vi "Write.Lookup.vi"(8 "error in":errorcluster, 10 "Name":string, 11 "Data Access API in":refnum<class "Plugin Data Access Engine.lvclass">) -> (0 "error out":errorcluster, 1 "Initial Values":dbl[](array[numeric]), 2 "Ref":T1, 3 "Data Access API out":refnum<class "Plugin Data Access Engine.lvclass">)   [LabVIEW 2023, in "Plugin Data Access Engine.lvlib" / "Plugin Data Access Engine.lvclass"]
uses:
  Plugin Data Access Engine.lvclass
  Types/Write.DVR.ctl
  Access Type Classes/Write/Write.lvclass
  Plugin Data Access Engine.lvclass/Plugin Data Access Engine.ctl
  Types/VS Channel Group Type.ctl
  Access Type Classes/Write/Write.lvclass/Write.ctl
  Access Type Classes/Write/Write.ReadValues.vi
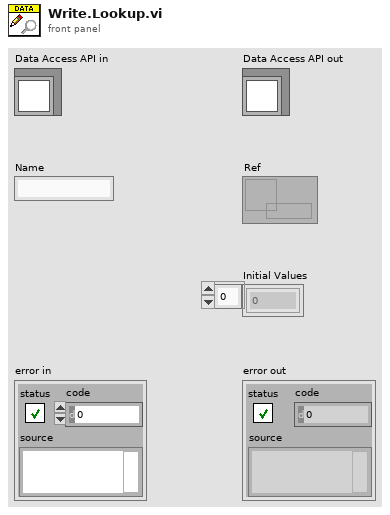
[diagram p1: front panel]
types:
  T1 = typedef "Plugin Data Access Engine.lvlib/Plugin Data Access Engine.lvclass/Write.DVR.ctl" = refnum<data-value>
  T2 = typedef "Plugin Data Access Engine.lvlib/Plugin Data Access Engine.lvclass/VS Channel Group Type.ctl" = enum16{"Output/Write", "Input/Read", "Input/ReadWrite"}
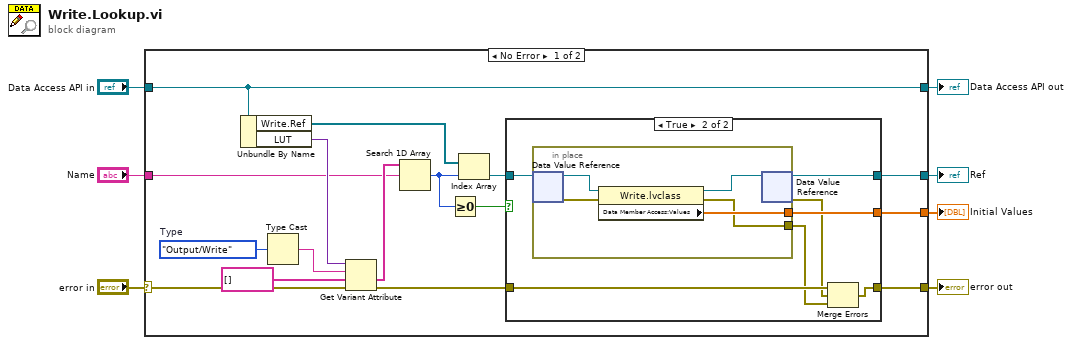
[diagram p0: block diagram]
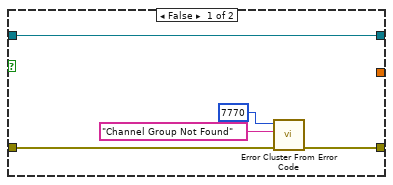
[diagram p2: hidden frame]
diagram:
  n1 = case shown="No Error" "error in" {
    selector: "error in" -> [w19 w42]
    tunnel: [w11 w42] -> w6
    tunnel: [w23 w41] -> w4
    tunnel: "Data Access API in" -> [w23 w41]
    tunnel: "Name" -> [w14 _]
    tunnel: [w10 _] -> w2
    tunnel: [w8 _] -> w1
    frame No Error {
      w16 = VS_Channel_Group_Type."Output/Write"  # Type
      n2 = Unbundle By Name(w23) -> ("Write.Ref"=w17:refnum<data-value>[], "LUT"=w22:variant)
      n3 = Type Cast(x=w16) -> (*(type *) &x=w21:string)  [unwired: 1 in]
      n4 = Get Variant Attribute(Variant=w22, name=w21, default value (empty Variant)=string[] [], error in=w19) -> (value=w18:string[], error out=w12:errorcluster)  [unwired: 2 out]
      n5 = Search 1D Array(1D array=w18, element=w14) -> (index of element=w15:i32)  [unwired: 1 in]
      n6 = Greater Or Equal To 0?(x=w15) -> (x >= 0?=w13:bool)
      n7 = Index Array(array=w17, index=w15) -> (element=w9:refnum<data-value>)
      n8 = case shown="True" w13 {
        tunnel: w12 -> [w28 w32]
        tunnel: [w27 w31] -> w11
        tunnel: [w24 w34] -> w10
        tunnel: w9 -> [w24 w35]
        tunnel: [_ w33] -> w8
        frame False {
          n9 = call <vilib>:"Error Cluster From Error Code.vi"("error in (no error)"=w28, "error message (\"\")"="Channel Group Not Found" ("error message (\"\")"), "error code (0)"=7770) -> ("error out"=w27:errorcluster)  [unwired: 6 in]
        }
        frame True {
          n10 = in-place {
            in-place-border: [w37] -> w33
            in-place-border: [w36] -> w29
            n11 = in-place-dvr #1(w35) -> (w40:refnum<class "Write.lvclass">, w39:errorcluster)
            n12 = property class="Write.lvclass"(reference=w40, error in=w39) -> (reference out=w38:refnum<class "Write.lvclass">, error out=w36:errorcluster, "Data Member Access:Values"=w37:dbl[])
            n13 = in-place-dvr #1(w38) -> (w34:refnum<data-value>, w30:errorcluster)
          }
          n14 = Merge Errors(w32, w30, w29) -> (w31:errorcluster)
        }
      }
    }
    frame Error {
    }
  }
  "error out" <- w6
  "Data Access API out" <- w4
  "Ref" <- w2
  "Initial Values" <- w1
